vi "waitOnIRQ.vi"(8 "error in (no error)":errorcluster, 10 "Timeout (ms)":i32, 11 "ModbusIRQs in":refnum<class "ModbusIRQs.lvclass">) -> (0 "error out":errorcluster, 1 "TimedOut":bool, 2 "IRQs":i32[](array[numeric]), 3 "ModbusIRQs out":refnum<class "ModbusIRQs.lvclass">)   [LabVIEW 2016, in "ModbusIRQs.lvclass"]
uses:
  ModbusIRQs.lvclass
  ModbusIRQs.lvclass/ModbusIRQs.ctl
  <vilib>/Utility/error.llb/Error Cluster From Error Code.vi
  <vilib>/RVI Host/nirviSupport.llb/nirviErrorClusterFromErrorCode.vi
  <vilib>/rvi/errors/niLvFpgaAdjustHostInterfaceError.vi
  <vilib>/rvi/interface/nirviMethod/nirviMethod.xnode
  <vilib>/rvi/interface/nirviMethod/StockFPGA_InlinedMethodWaitForMultipleIRQ.vi
  <vilib>/FPGAPlugInAG/Dynamic/niLvFpga_WaitOnIrq_Dynamic.vi
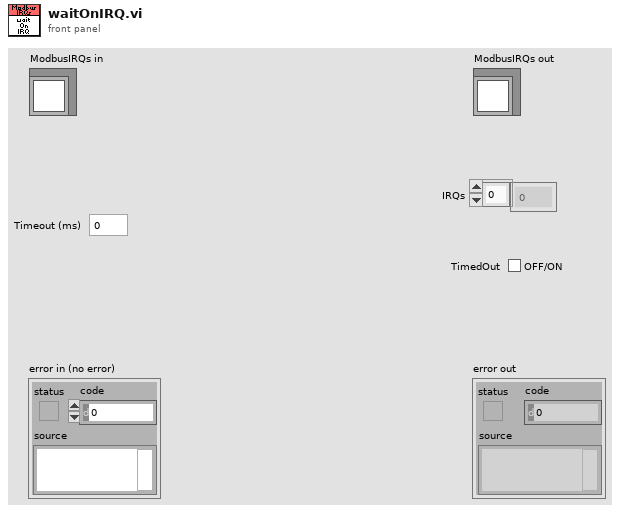
[diagram p1: front panel]
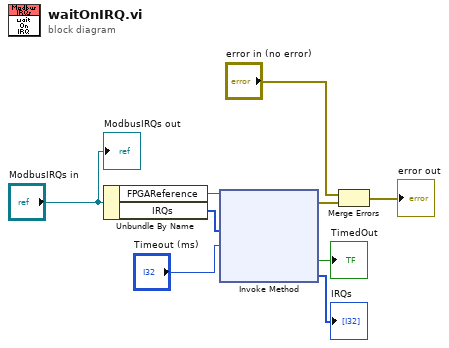
[diagram p0: block diagram]
diagram:
  n1 = Unbundle By Name("ModbusIRQs in") -> ("FPGAReference"=w9:refnum<k20>, "IRQs"=w8:i32[])
  n2 = xnode "Invoke Method"("FPGA VI Reference In"=w9, "IRQ Number(s)"=w8, "Timeout (ms)"="Timeout (ms)") -> ("error out"=w3:errorcluster, "Timed Out"=→"TimedOut":bool, "IRQ(s) Asserted"=→"IRQs":i32[])  [unwired: 1 in, 1 out]
  n3 = Merge Errors("error in (no error)", w3) -> (→"error out":errorcluster)
  "ModbusIRQs out" <- "ModbusIRQs in"
